vi "DetectCollisionImproved.vi"(0 "ball":dbl[](array[numeric]), 4 "Goal":dbl[](array[numeric]), 5 "our_robots":T1[](array[typedef]), 6 "Initial State":dbl[](array[numeric]), 7 "enemy_robots":T1[](array[typedef]), 8 "Is not first robot?":bool, 9 "element being analyzed":dbl[](array[numeric]), 10 "element already in path":dbl[](array[numeric]), 11 "Robot in":T1) -> (2 "Is there colision?":bool)   [LabVIEW 2017]
uses:
  Core/AI Robot.ctl
  Intel/Functions Enum.ctl
  Intel/AttackerStates.ctl
  PathDests.ctl
  PathDest.ctl
  <vilib>/Analysis/_algsub.llb/Real Vector Norm.vi
  <vilib>/Analysis/baseanly.llb/Real Dot Product.vi
  <vilib>/Analysis/NI_AALBase.lvlib
  <vilib>/Analysis/NI_AALPro.lvlib
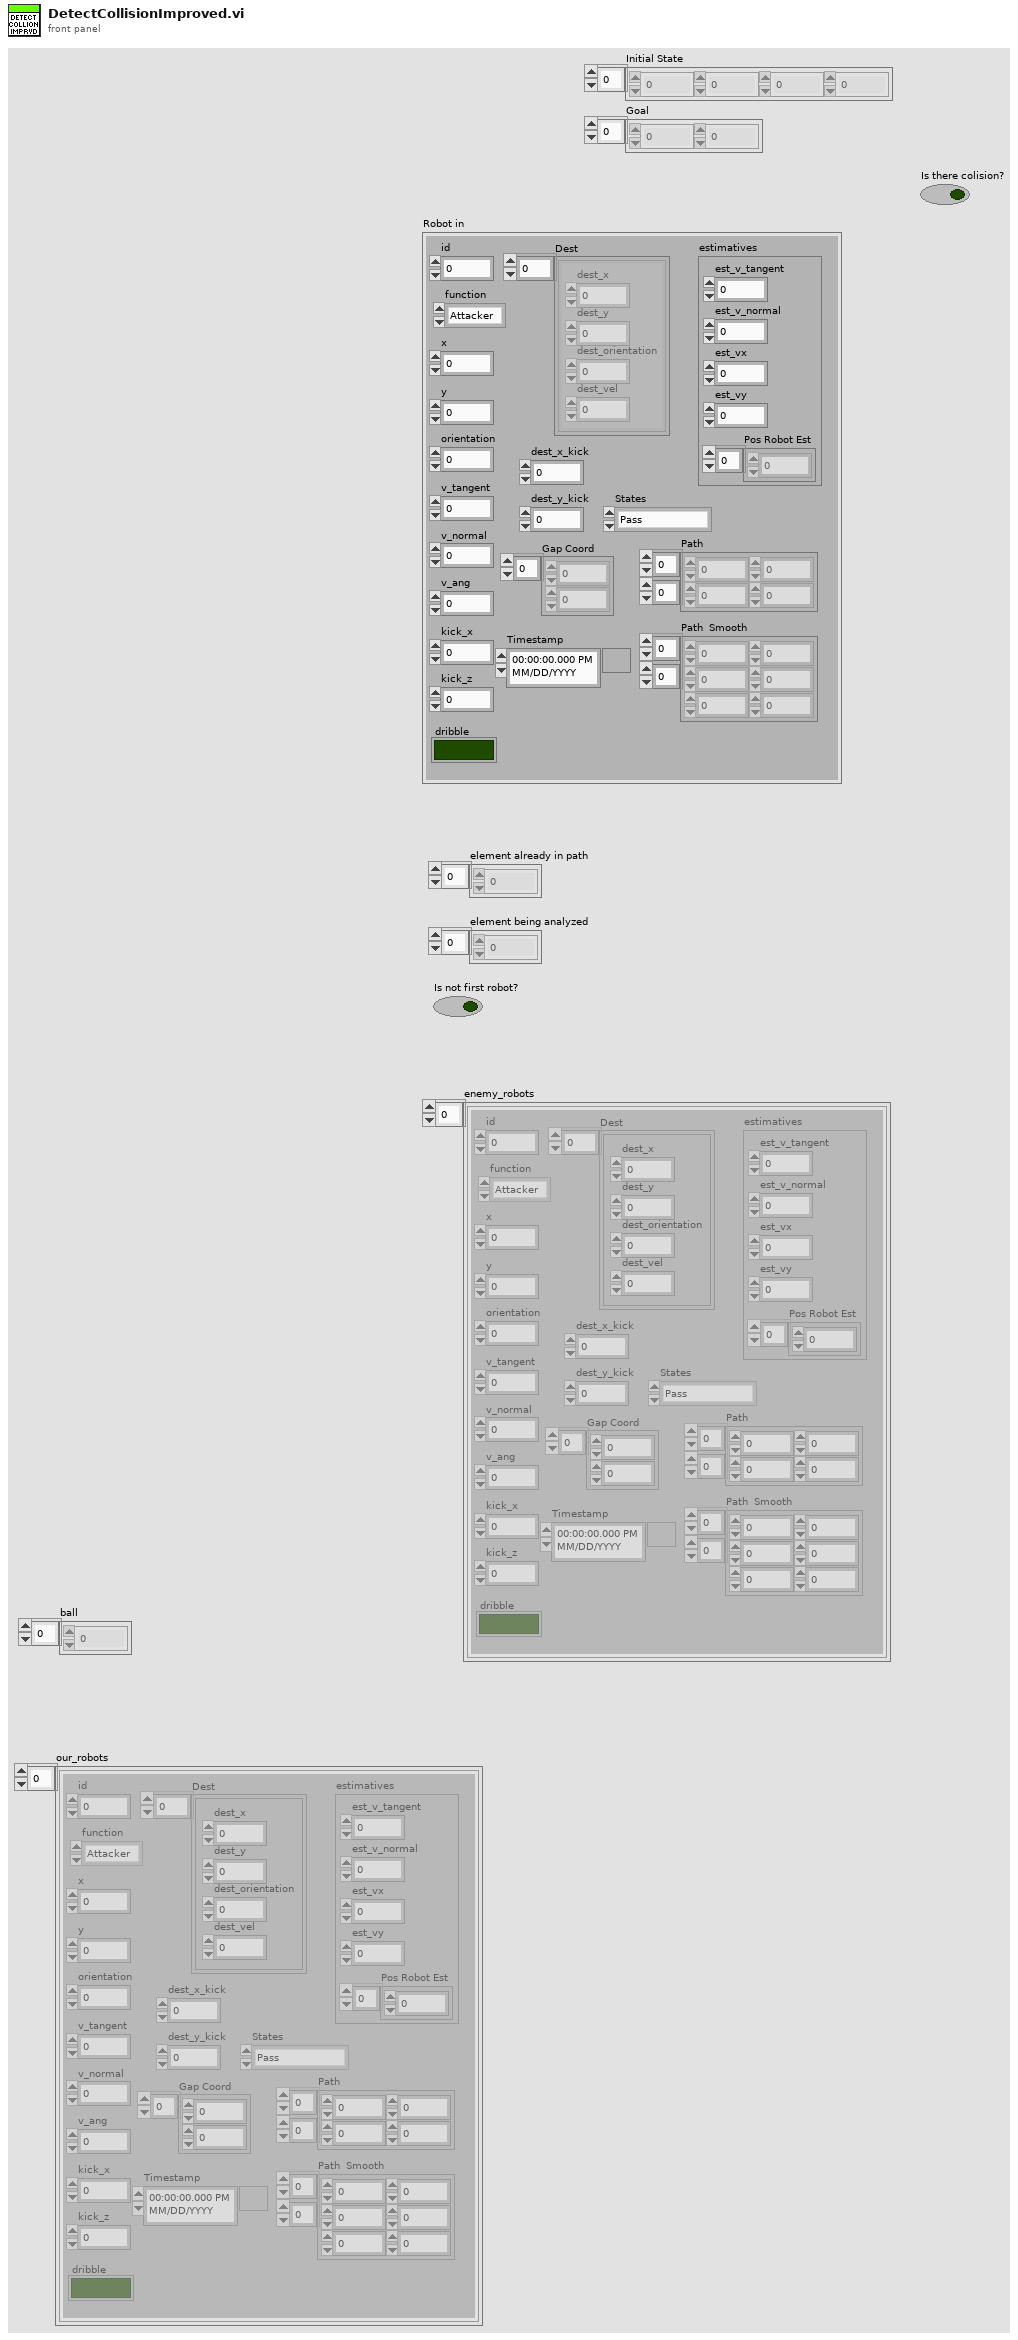
[diagram p1: front panel]
types:
  T1 = typedef "AI Robot.ctl" = cluster{"id":u32, "function":T2, "x":dbl, "y":dbl, "orientation":dbl, "v_tangent":dbl, "v_normal":dbl, "v_ang":dbl, "kick_x":dbl, "kick_z":dbl, "dribble":bool, "Timestamp":timestamp, "estimatives":cluster{"est_v_tangent":dbl, "est_v_normal":dbl, "est_vx":dbl, "est_vy":dbl, "Pos Robot Est":dbl[]}, "dest_x_kick":dbl, "dest_y_kick":dbl, "Gap Coord":dbl[], "States":T3, "Path ":dbl[][], "Path  Smooth":dbl[][], "Dest":T4}
  T2 = typedef "Functions Enum.ctl" = enum16{"Attacker", "Goalie", "Defender", "Striker", "Goto 0", "Dummy", "Kicker", "ZigZag"}
  T3 = typedef "AttackerStates.ctl" = enum16{"Pass", "GoToTangent", "BallGetting", "GoToKick", ""}
  T4 = typedef "PathDests.ctl" = T5[]
  T5 = typedef "PathDest.ctl" = cluster{"dest_x":dbl, "dest_y":dbl, "dest_orientation":dbl, "dest_vel":dbl}
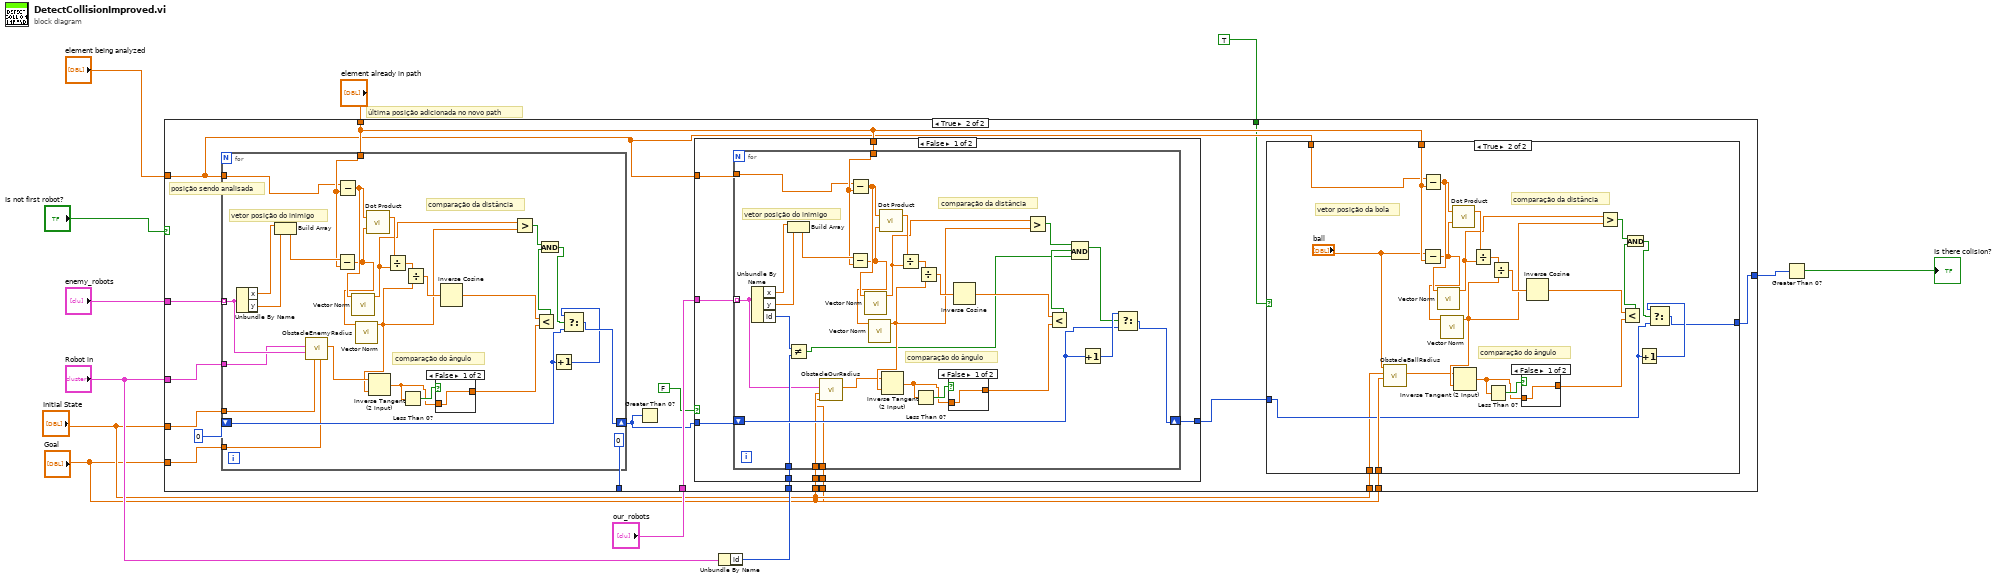
[diagram p0: block diagram]
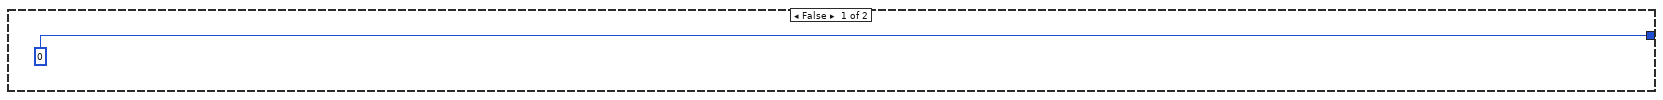
[diagram p2: hidden frame]
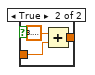
[diagram p4: hidden frame]
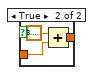
[diagram p5: hidden frame]
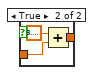
[diagram p7: hidden frame]
diagram:
  # "última posição adicionada no novo path"
  n1 = Unbundle By Name("Robot in") -> ("id"=w4:u32)
  n2 = case shown="True" "Is not first robot?" {
    tunnel: "enemy_robots" -> [_ w32]
    tunnel: "element being analyzed" -> [_ w19]
    tunnel: "element already in path" -> [_ w20]
    tunnel: [0 w16] -> w12
    tunnel: "Robot in" -> [_ w30]
    tunnel: "Initial State" -> [_ w29]
    tunnel: "Goal" -> [_ w28]
    tunnel: 0 -> [_ _]
    tunnel: "our_robots" -> [_ w27]
    tunnel: w4 -> [_ w26]
    tunnel: "Initial State" -> [_ w24]
    tunnel: "Goal" -> [_ w23]
    tunnel: "Initial State" -> [_ w18]
    tunnel: "Goal" -> [_ w17]
    tunnel: TRUE -> [_ w15]
    frame False {
    }
    frame True {
      # "posição sendo analisada"
      n3 = for {
        tunnel: w32 -> [w108] mode=indexing
        shift-right: [w118] -> w25
        shift-left: 0 -> [w116]
        tunnel: w19 -> [w125]
        tunnel: w20 -> [w126]
        tunnel: w30 -> [w107]
        tunnel: w29 -> [w106]
        tunnel: w28 -> [w105]
        # "comparação do ângulo"
        # "comparação da distância"
        # "vetor posição do inimigo"
        n4 = Unbundle By Name(w108) -> ("x"=w129:dbl, "y"=w128:dbl)
        n5 = Build Array(w129, w128) -> (w127:dbl[])
        n6 = call "ObstacleEnemyRadius.vi"("Goal"=w105, "Initial State"=w106, "Robot enemy"=w108, "Robot in"=w107) -> ("obstacle enemy radius"=w104:dbl)  [unwired: 7 in]
        n7 = Subtract(x=w127, y=w126) -> (x-y=w119:dbl[])
        n8 = Subtract(x=w125, y=w126) -> (x-y=w123:dbl[])
        n9 = call-poly <vilib>:"Vector Norm.vi"("Input Vector"=w123) -> ("norm"=w115:dbl)  [unwired: 9 in, 1 out]
        n10 = call-poly <vilib>:"Vector Norm.vi"("Input Vector"=w119) -> ("norm"=w103:dbl)  [unwired: 9 in, 1 out]
        n11 = call-poly <vilib>:"Dot Product.vi"("Y Vector"=w119, "X Vector"=w123) -> ("X * Y"=w124:dbl)  [unwired: 1 out]
        n12 = Inverse Tangent (2 Input)(1:w103, 2:w104) -> (0:w110:dbl)
        n13 = Divide(x=w124, y=w115) -> (x/y=w122:dbl)
        n14 = Less Than 0?(x=w110) -> (x < 0?=w111:bool)
        n15 = Divide(x=w122, y=w103) -> (x/y=w121:dbl)
        n16 = case shown="False" w111 {
          tunnel: w110 -> [w130 w132]
          tunnel: [w130 w131] -> w109
          frame False {
          }
          frame True {
            n17 = Add(x=3.141592653589793, y=w132) -> (x+y=w131:dbl)
          }
        }
        n18 = Inverse Cosine(1:w121) -> (0:w120:dbl)
        n19 = Greater?(x=w115, y=w103) -> (0:w114:bool)
        n20 = Less?(x=w120, y=w109) -> (x < y?=w113:bool)
        n21 = And(x=w114, y=w113) -> (x .and. y?=w112:bool)
        n22 = Increment(x=w116) -> (x+1=w117:i32)
        n23 = Select(t=w117, s=w112, f=w116) -> (s? t:f=w118:i32)
      }
      n24 = Greater Than 0?(x=w25) -> ()  [unwired: 1 out]
      n25 = case shown="False" FALSE {
        tunnel: w25 -> [w68 w102]
        tunnel: w27 -> [w67 _]
        tunnel: w20 -> [w66 _]
        tunnel: w19 -> [w65 _]
        tunnel: w26 -> [w64 _]
        tunnel: [w63 w102] -> w21
        tunnel: w24 -> [w62 _]
        tunnel: w23 -> [w61 _]
        frame False {
          n26 = for {
            tunnel: w67 -> [w72] mode=indexing
            shift-right: [w86] -> w63
            shift-left: w68 -> [w77]
            tunnel: w65 -> [w93]
            tunnel: w66 -> [w94]
            tunnel: w64 -> [w74]
            tunnel: w62 -> [w71]
            tunnel: w61 -> [w70]
            # "comparação do ângulo"
            # "comparação da distância"
            # "vetor posição do inimigo"
            n27 = Unbundle By Name(w72) -> ("x"=w97:dbl, "y"=w96:dbl, "id"=w75:u32)
            n28 = Build Array(w97, w96) -> (w95:dbl[])
            n29 = Not Equal?(x=w75, y=w74) -> (x != y?=w73:bool)
            n30 = call "ObstacleOurRadius.vi"("Goal"=w70, "Initial State"=w71, "other robot"=w72) -> ("obstacle enemy radius"=w69:dbl)  [unwired: 8 in]
            n31 = Subtract(x=w95, y=w94) -> (x-y=w87:dbl[])
            n32 = Subtract(x=w93, y=w94) -> (x-y=w91:dbl[])
            n33 = call-poly <vilib>:"Vector Norm.vi"("Input Vector"=w91) -> ("norm"=w84:dbl)  [unwired: 9 in, 1 out]
            n34 = call-poly <vilib>:"Vector Norm.vi"("Input Vector"=w87) -> ("norm"=w78:dbl)  [unwired: 9 in, 1 out]
            n35 = call-poly <vilib>:"Dot Product.vi"("Y Vector"=w87, "X Vector"=w91) -> ("X * Y"=w92:dbl)  [unwired: 1 out]
            n36 = Inverse Tangent (2 Input)(1:w78, 2:w69) -> (0:w80:dbl)
            n37 = Divide(x=w92, y=w84) -> (x/y=w90:dbl)
            n38 = Less Than 0?(x=w80) -> (x < 0?=w81:bool)
            n39 = Divide(x=w90, y=w78) -> (x/y=w89:dbl)
            n40 = case shown="False" w81 {
              tunnel: w80 -> [w98 w100]
              tunnel: [w98 w99] -> w79
              frame False {
              }
              frame True {
                n41 = Add(x=3.141592653589793, y=w100) -> (x+y=w99:dbl)
              }
            }
            n42 = Inverse Cosine(1:w89) -> (0:w88:dbl)
            n43 = Greater?(x=w84, y=w78) -> (0:w83:bool)
            n44 = Less?(x=w88, y=w79) -> (x < y?=w82:bool)
            n45 = Compound Arithmetic op=AND(w83, w82, w73) -> (w76:bool)
            n46 = Increment(x=w77) -> (x+1=w85:i32)
            n47 = Select(t=w85, s=w76, f=w77) -> (s? t:f=w86:i32)
          }
        }
        frame True {
        }
      }
      n48 = case shown="True" w15 {
        tunnel: w21 -> [w33 w36]
        tunnel: w20 -> [_ w41]
        tunnel: w19 -> [_ w40]
        tunnel: w18 -> [_ w34]
        tunnel: w17 -> [_ w37]
        tunnel: [w33 w35] -> w16
        frame False {
        }
        frame True {
          # "comparação do ângulo"
          # "comparação da distância"
          # "vetor posição da bola"
          n49 = call "ObstacleBallRadius.vi"("Goal"=w37, "Initial State"=w34, "ball"="ball") -> ("obstacle enemy radius"=w39:dbl)  [unwired: 8 in]
          n50 = Subtract(x="ball", y=w41) -> (x-y=w51:dbl[])
          n51 = Subtract(x=w40, y=w41) -> (x-y=w55:dbl[])
          n52 = call-poly <vilib>:"Vector Norm.vi"("Input Vector"=w55) -> ("norm"=w49:dbl)  [unwired: 9 in, 1 out]
          n53 = call-poly <vilib>:"Vector Norm.vi"("Input Vector"=w51) -> ("norm"=w42:dbl)  [unwired: 9 in, 1 out]
          n54 = call-poly <vilib>:"Dot Product.vi"("Y Vector"=w51, "X Vector"=w55) -> ("X * Y"=w56:dbl)  [unwired: 1 out]
          n55 = Inverse Tangent (2 Input)(1:w42, 2:w39) -> (0:w44:dbl)
          n56 = Divide(x=w56, y=w49) -> (x/y=w54:dbl)
          n57 = Less Than 0?(x=w44) -> (x < 0?=w45:bool)
          n58 = Divide(x=w54, y=w42) -> (x/y=w53:dbl)
          n59 = case shown="False" w45 {
            tunnel: w44 -> [w57 w59]
            tunnel: [w57 w58] -> w43
            frame False {
            }
            frame True {
              n60 = Add(x=3.141592653589793, y=w59) -> (x+y=w58:dbl)
            }
          }
          n61 = Inverse Cosine(1:w53) -> (0:w52:dbl)
          n62 = Greater?(x=w49, y=w42) -> (0:w48:bool)
          n63 = Less?(x=w52, y=w43) -> (x < y?=w47:bool)
          n64 = And(x=w48, y=w47) -> (x .and. y?=w46:bool)
          n65 = Increment(x=w36) -> (x+1=w50:i32)
          n66 = Select(t=w50, s=w46, f=w36) -> (s? t:f=w35:i32)
        }
      }
    }
  }
  n67 = Greater Than 0?(x=w12) -> (x > 0?=→"Is there colision?":bool)
